vi "GetFlatSequenceFrames.vi"(5 "FlatSequence in":refnum<class "FlatSequence.lvclass">, 6 "error in":errorcluster, 9 "VI Interpreter in":refnum<class "VI Interpreter.lvclass">) -> (0 "error out":errorcluster, 3 "VI Interpreter out":refnum<class "VI Interpreter.lvclass">, 4 "FlatSequence out":refnum<class "FlatSequence.lvclass">)   [LabVIEW 2014, in "Raspberry Pi Compatible Compiler for LabVIEW.lvlib" / "VI Interpreter.lvclass"]
uses:
  VI Interpreter.lvclass
  FlatSequence/FlatSequence.lvclass
  FlatSequenceFrame/FlatSequenceFrame.lvclass/FlatSequenceFrame.ctl
  FlatSequence/FlatSequence.lvclass/FlatSequence.ctl
  FlatSequenceFrame/FlatSequenceFrame.lvclass
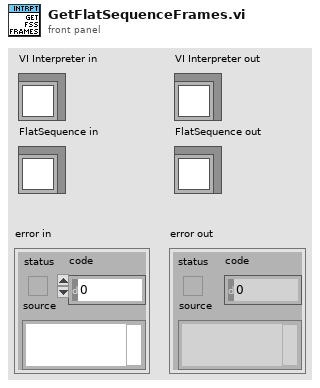
[diagram p1: front panel]
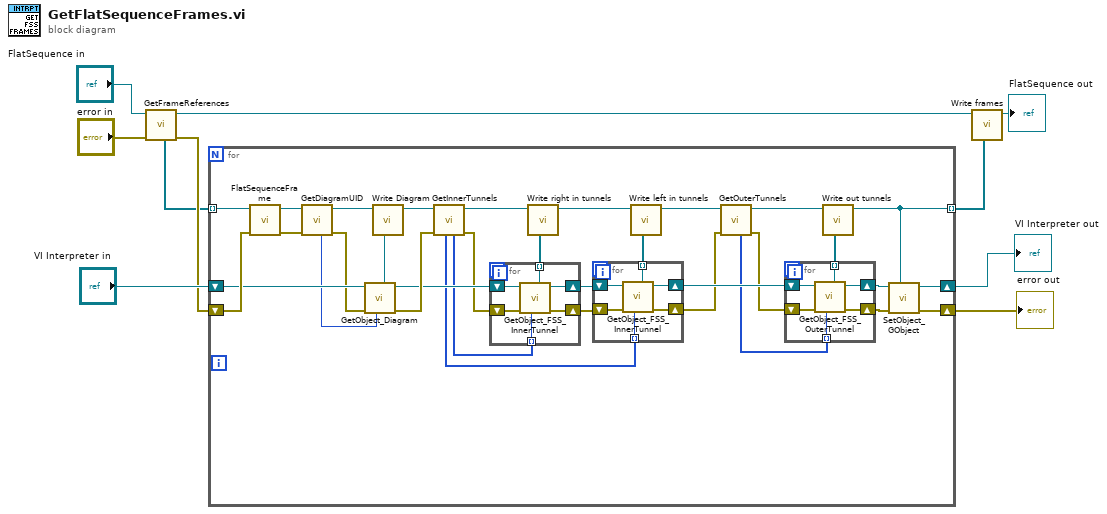
[diagram p0: block diagram]
diagram:
  n1 = call "GetFrameReferences.vi"("error in"="error in", "FlatSequence in"="FlatSequence in") -> ("error out"=w5:errorcluster, "FlatSequence out"=w3:refnum<class "FlatSequence.lvclass">, "Frames[]"=w4:refnum<vi>[])  [unwired: 5 in]
  n2 = for {
    shift-right: [w43] -> w10
    shift-left: "VI Interpreter in" -> [w37]
    tunnel: w4 -> [w40] mode=indexing
    shift-right: [w42] -> w9
    shift-left: w5 -> [w41]
    tunnel: [w20] -> w2 mode=indexing
    n3 = call "FlatSequenceFrame.vi"("error in"=w41, "reference"=w40) -> ("error out"=w38:errorcluster, "Flat Sequence Frame out"=w39:refnum<class "FlatSequenceFrame.lvclass">)  [unwired: 8 in]
    n4 = call-dynamic "GetDiagramUID.vi"("error in"=w38, "FlatSequenceFrame in"=w39) -> ("error out"=w36:errorcluster, "FlatSequenceFrame out"=w35:refnum<class "FlatSequenceFrame.lvclass">, "Diagram.UID"=w33:i32)  [unwired: 5 in]
    n5 = call "GetObject_Diagram.vi"("UID"=w33, "error in"=w36, "VI Interpreter in"=w37) -> ("error out"=w31:errorcluster, "VI Interpreter out"=w30:refnum<class "VI Interpreter.lvclass">, "Diagram"=w34:refnum<class "Diagram.lvclass">)  [unwired: 3 in, 1 out]
    n6 = call "Write Diagram.vi"("Diagram.lvclass"=w34, "FlatSequenceFrame in"=w35) -> ("FlatSequenceFrame out"=w32:refnum<class "FlatSequenceFrame.lvclass">)  [unwired: 7 in]
    n7 = call-dynamic "GetInnerTunnels.vi"("error in"=w31, "FlatSequenceFrame in"=w32) -> ("error out"=w29:errorcluster, "FlatSequenceFrame out"=w23:refnum<class "FlatSequenceFrame.lvclass">, "right inside"=w25:i32[], "left inside"=w26:i32[])  [unwired: 4 in]
    n8 = for {
      shift-right: [w57] -> w28
      shift-left: w30 -> [w61]
      tunnel: w25 -> [w60] mode=indexing
      shift-right: [w58] -> w27
      shift-left: w29 -> [w59]
      tunnel: [w56] -> w24 mode=indexing
      n9 = call "GetObject_FSS_InnerTunnel.vi"("UID"=w60, "error in"=w59, "VI Interpreter in"=w61) -> ("error out"=w58:errorcluster, "VI Interpreter out"=w57:refnum<class "VI Interpreter.lvclass">, "Tunnel"=w56:refnum<class "FlatSequenceInnerTunnel.lvclass">)  [unwired: 3 in, 1 out]
    }
    n10 = call "Write right in tunnels.vi"("right in tunnels"=w24, "FlatSequenceFrame in"=w23) -> ("FlatSequenceFrame out"=w22:refnum<class "FlatSequenceFrame.lvclass">)  [unwired: 7 in]
    n11 = for {
      shift-right: [w52] -> w17
      shift-left: w28 -> [w55]
      shift-right: [w53] -> w13
      shift-left: w27 -> [w54]
      tunnel: [w51] -> w21 mode=indexing
      tunnel: w26 -> [w50] mode=indexing
      n12 = call "GetObject_FSS_InnerTunnel.vi"("UID"=w50, "error in"=w54, "VI Interpreter in"=w55) -> ("error out"=w53:errorcluster, "VI Interpreter out"=w52:refnum<class "VI Interpreter.lvclass">, "Tunnel"=w51:refnum<class "FlatSequenceInnerTunnel.lvclass">)  [unwired: 3 in, 1 out]
    }
    n13 = call "Write left in tunnels.vi"("left in tunnels"=w21, "FlatSequenceFrame in"=w22) -> ("FlatSequenceFrame out"=w15:refnum<class "FlatSequenceFrame.lvclass">)  [unwired: 7 in]
    n14 = call-dynamic "GetOuterTunnels.vi"("error in"=w13, "FlatSequenceFrame in"=w15) -> ("error out"=w12:errorcluster, "FlatSequenceFrame out"=w14:refnum<class "FlatSequenceFrame.lvclass">, "outside tunnels"=w11:i32[])  [unwired: 5 in]
    n15 = for {
      shift-right: [w46] -> w19
      shift-left: w17 -> [w49]
      shift-right: [w47] -> w18
      shift-left: w12 -> [w48]
      tunnel: [w45] -> w16 mode=indexing
      tunnel: w11 -> [w44] mode=indexing
      n16 = call "GetObject_FSS_OuterTunnel.vi"("UID"=w44, "error in"=w48, "VI Interpreter in"=w49) -> ("error out"=w47:errorcluster, "VI Interpreter out"=w46:refnum<class "VI Interpreter.lvclass">, "Tunnel"=w45:refnum<class "FlatSequenceOuterTunnel.lvclass">)  [unwired: 3 in, 1 out]
    }
    n17 = call "Write out tunnels.vi"("out tunnels"=w16, "FlatSequenceFrame in"=w14) -> ("FlatSequenceFrame out"=w20:refnum<class "FlatSequenceFrame.lvclass">)  [unwired: 7 in]
    n18 = call "SetObject_GObject.vi"("GObject"=w20, "error in"=w18, "VI Interpreter in"=w19) -> ("error out"=w42:errorcluster, "VI Interpreter out"=w43:refnum<class "VI Interpreter.lvclass">)  [unwired: 5 in]
  }
  "error out" <- w9
  "VI Interpreter out" <- w10
  n19 = call "Write frames.vi"("frames"=w2, "FlatSequence in"=w3) -> ("FlatSequence out"=→"FlatSequence out":refnum<class "FlatSequence.lvclass">)  [unwired: 7 in]
